vi "Facade.vi"(0 "Data In":T7, 2 "Display State In":T2={"Graph Visible Items"={"Plot Legend"=FALSE, "Scale Legend"=FALSE, "Graph Palette"=FALSE, "Cursor Legend"=FALSE, "X Scrollbar"=FALSE}, "View Table"=FALSE, "Table Visible Items"={"Vertical Scrollbar"=FALSE, "Horizontal Scrollbar"=FALSE, "Row Headers"=FALSE, "Column Headers"=FALSE, "Vertical Lines"=FALSE, "Horizontal Lines"=FALSE}, "Header Font"={"Font Name"="", "Size"=0, "Bold"=FALSE, "Italic"=FALSE, "Underline"=FALSE, "Strikeout"=FALSE, "Color"=0}, "Cell Font"={"Font Name"="", "Size"=0, "Bold"=FALSE, "Italic"=FALSE, "Underline"=FALSE, "Strikeout"=FALSE, "Color"=0}, "Description and Tip..."={"Description"="", "Tip"=""}, "Moveable Splitter Position"=0, "Measurement Cursor Configuration"={"XY"={"enable XY"=FALSE, "Position (X)"=[], "Type"=enum."Absolute", "Y reference"=0.0, "color"=0}, "band"={"enable band"=FALSE, "B1"=0.0, "B2"=0.0, "Fixed bandwidth (B2-B1)"=0.0, "B1 color"=0, "B2 color"=0}, "harmonic"={"enable harmonics"=FALSE, "X reference (1X)"=0.0, "Maximum"=0, "Subset"=enum."All", "1X color"=0, "MX color"=0}, "sideband"={"enable sideband"=FALSE, "X center (C)"=0.0, "Sidebands"=0, "X spacing (s)"=0.0, "Center color"=0, "Sideband color"=0}}, "Cursors"={"List"=[], "Tags"=[]}, "X Increment"=0.0, "X Scale"={"Label Visible"=FALSE, "Label Text"="", "Mapping Mode"=0, "Format String"=""}, "Y Scale"={"Label Visible"=FALSE, "Label Text"="", "Mapping Mode"=0, "Format String"=""}, "Colors"={"background"=16777215, "major grid"=8355711, "minor grid"=12632256, "font"=0}, "desired spectrum view"={"scaling"={"linear/dB"=enum."no change", "dB reference"=0.0, "power/magnitude"=enum."no change", "view"=enum."no change"}, "spectral density"=enum."no change"}, "Plot Color Wheel"=[3381759, 32768, 982784, 4375295, 13827953, 13457919, 16757522, 4343295, 16728758, 12095254], "Plots"=[], "registered user events"=variant, "Lock 1X to Peak"=FALSE, "spectrum component"=32, "phase spectrum view"={"desired units"=0, "desired wrapping"=4}} {"phase spectrum view"."desired wrapping" items=["No change", "Unwrap", "Wrap: -360 to 0", "Wrap: -270 to 90", "Wrap: -180 to 180", "Wrap: -90 to 270", "Wrap: 0 to 360", "Wrap: custom range"]; "phase spectrum view"."desired units" items=["No change", "Radians", "Degrees", "Cycles"]; "spectrum component" items=["Magnitude^2"=37, "Magnitude"=32, "Phase"=33, "Real"=34, "Imaginary"=35, "Coherence"=36, "Unknown"=99]; "Y Scale"."Mapping Mode" items=["Linear", "Logarithmic", "dB"]; "X Scale"."Mapping Mode" items=["Linear", "Logarithmic"]}, 3 "Container State":T6) -> (6 "Data Out":T7, 7 "Display State Out":T2={"Graph Visible Items"={"Plot Legend"=FALSE, "Scale Legend"=FALSE, "Graph Palette"=FALSE, "Cursor Legend"=FALSE, "X Scrollbar"=FALSE}, "View Table"=FALSE, "Table Visible Items"={"Vertical Scrollbar"=FALSE, "Horizontal Scrollbar"=FALSE, "Row Headers"=FALSE, "Column Headers"=FALSE, "Vertical Lines"=FALSE, "Horizontal Lines"=FALSE}, "Header Font"={"Font Name"="", "Size"=0, "Bold"=FALSE, "Italic"=FALSE, "Underline"=FALSE, "Strikeout"=FALSE, "Color"=0}, "Cell Font"={"Font Name"="", "Size"=0, "Bold"=FALSE, "Italic"=FALSE, "Underline"=FALSE, "Strikeout"=FALSE, "Color"=0}, "Description and Tip..."={"Description"="", "Tip"=""}, "Moveable Splitter Position"=0, "Measurement Cursor Configuration"={"XY"={"enable XY"=FALSE, "Position (X)"=[], "Type"=enum."Absolute", "Y reference"=0.0, "color"=0}, "band"={"enable band"=FALSE, "B1"=0.0, "B2"=0.0, "Fixed bandwidth (B2-B1)"=0.0, "B1 color"=0, "B2 color"=0}, "harmonic"={"enable harmonics"=FALSE, "X reference (1X)"=0.0, "Maximum"=0, "Subset"=enum."All", "1X color"=0, "MX color"=0}, "sideband"={"enable sideband"=FALSE, "X center (C)"=0.0, "Sidebands"=0, "X spacing (s)"=0.0, "Center color"=0, "Sideband color"=0}}, "Cursors"={"List"=[], "Tags"=[]}, "X Increment"=0.0, "X Scale"={"Label Visible"=FALSE, "Label Text"="", "Mapping Mode"=0, "Format String"=""}, "Y Scale"={"Label Visible"=FALSE, "Label Text"="", "Mapping Mode"=0, "Format String"=""}, "Colors"={"background"=16777215, "major grid"=8355711, "minor grid"=12632256, "font"=0}, "desired spectrum view"={"scaling"={"linear/dB"=enum."no change", "dB reference"=0.0, "power/magnitude"=enum."no change", "view"=enum."no change"}, "spectral density"=enum."no change"}, "Plot Color Wheel"=[3381759, 32768, 982784, 4375295, 13827953, 13457919, 16757522, 4343295, 16728758, 12095254], "Plots"=[], "registered user events"=variant, "Lock 1X to Peak"=FALSE, "spectrum component"=32, "phase spectrum view"={"desired units"=0, "desired wrapping"=4}} {"phase spectrum view"."desired wrapping" items=["No change", "Unwrap", "Wrap: -360 to 0", "Wrap: -270 to 90", "Wrap: -180 to 180", "Wrap: -90 to 270", "Wrap: 0 to 360", "Wrap: custom range"]; "phase spectrum view"."desired units" items=["No change", "Radians", "Degrees", "Cycles"]; "spectrum component" items=["Magnitude^2"=37, "Magnitude"=32, "Phase"=33, "Real"=34, "Imaginary"=35, "Coherence"=36, "Unknown"=99]; "Y Scale"."Mapping Mode" items=["Linear", "Logarithmic", "dB"]; "X Scale"."Mapping Mode" items=["Linear", "Logarithmic"]}, 8 "Action":T1)   [LabVIEW 2017, in "Spectrum with Cursors.xctl"]
doc: "This is the facade VI for the Spectral Graph with Measurement Cursors XControl.\nThe facade VI is only used within the context of the XControl."
uses:
  <vilib>/addons/_XControls/Spectrum with Cursors/Spectrum with Cursors.xctl
  <vilib>/addons/_XControls/Spectrum with Cursors/Controls/Data.ctl
  <vilib>/addons/_NISVFA/_Shared subVIs/Data Objects/Data/Data.lvclass
  <vilib>/_xctls/Container State.ctl
  <vilib>/addons/_XControls/Spectrum with Cursors/Controls/State.ctl
  <vilib>/Utility/miscctls.llb/LVFontTypeDef.ctl
  <vilib>/addons/_XControls/Spectrum with Cursors/Controls/Measurement Cursor Configuration.ctl
  <vilib>/addons/_NISVFA/_Shared subVIs/Controls/NI Spectrum Component.ctl
  <vilib>/_xctls/Action.ctl
  <vilib>/addons/_NISVFA/_Shared subVIs/Data Objects/Data/Data.lvclass/Data.ctl
  <vilib>/addons/_XControls/Spectrum with Cursors/Controls/Refnums Typedef.ctl
  <vilib>/addons/_NISVFA/_Shared subVIs/Data Objects/Y (DBL)/Y (N Ch).lvclass/Y (N Ch).ctl
  <vilib>/addons/_XControls/Spectrum with Cursors/Controls/Spectrum XControl Events.ctl
  <vilib>/Utility/miscctls.llb/LVForegroundBackgroundColorsTypeDef.ctl
  <vilib>/addons/_NISVFA/_Shared subVIs/Data Objects/Data/Read Channel Count.vi
  <vilib>/addons/_NISVFA/_Shared subVIs/Data Objects/Y (DBL)/SV Convert Spectra to Data Object.vi
  <vilib>/addons/_NISVFA/_Spectrum Processing/SVFA Get Spectrum Subset (1 Ch).vi
  <vilib>/addons/_NISVFA/_Spectrum Processing/SVFA Spectrum Peak Search (1 Ch).vi
  <vilib>/addons/_NISVFA/_Shared subVIs/Data Objects/Data/Read Data Attributes.vi
  <vilib>/addons/_NISVFA/_Shared subVIs/Data Objects/subVIs/Get Channel Count.vi
  <vilib>/addons/_NISVFA/_Shared subVIs/Common/sv_Get NI Property Name String.vi
  <vilib>/addons/_NISVFA/_Shared subVIs/Data Objects/Data/Write Data Attributes.vi
  <vilib>/addons/_NISVFA/_Shared subVIs/Data Objects/subVIs/Set Channel Count.vi
  <vilib>/addons/_NISVFA/_Shared subVIs/Common/svc_Spectrum Units.vi
  <vilib>/addons/_NISVFA/_Spectrum Processing/subVIs/svfa_Spectrum Peak Search.vi
  <vilib>/addons/_NISVFA/_Spectrum Processing/subVIs/svfa_Peak Rough Search Indices.vi
  <vilib>/addons/_NISVFA/_Shared subVIs/Data Objects/Y (DBL)/Y (N Ch).lvclass
  C:/Program Files (x86)/National Instruments/LabVIEW 2017/vi.lib/addons/_NISVFA/_Shared subVIs/Data Objects/Data/Data.lvclass
  <vilib>/addons/_NISVFA/_Spectrum Processing/SVFA Phase Unit Conversion (N Ch).vi
  <vilib>/addons/_NISVFA/_Spectrum Processing/SVFA Wrap or Unwrap Phase (N Ch).vi
  <vilib>/addons/_NISVFA/_Shared subVIs/Common/svc_Caller VI Returned in Error Source.vi
  <vilib>/addons/_NISVFA/_Shared subVIs/Common/svc_Get Weighting Enum and Labels.vi
  <vilib>/addons/_NISVFA/_Shared subVIs/Common/svc_Unit Label Lexical Class.vi
  <vilib>/addons/_NISVFA/_Shared subVIs/Common/svc_Engineering Units to Unit Label.vi
  <vilib>/addons/_NISVFA/_Shared subVIs/Common/svc_Format Value (DBL).vi
  <vilib>/addons/_NISVFA/_Spectrum Processing/subVIs/svfa_Three Finger Peak Search.vi
  <vilib>/addons/_NISVFA/_Shared subVIs/Common/svc_Build Unit Label for Frequency Range.vi
  <vilib>/addons/_NISVFA/_Shared subVIs/Common/svc_Convert Frequency to Frequency String.vi
  <vilib>/addons/_NISVFA/_Shared subVIs/Common/svc_Check Frequency Range in Spectrum.vi
  <vilib>/addons/_NISVFA/_Spectrum Processing/SVFA Unit Conversion (N Ch).vi
  <vilib>/addons/_NISVFA/_Shared subVIs/Spectrum Info/sv_Convert Spectrum Info to Variant Attributes.vi
  <vilib>/addons/_NISVFA/_Shared subVIs/Data Objects/Y (DBL)/Write Channels Array.vi
  <vilib>/_xctls/XControlSupport.lvlib
panel:
  out "plot names":string[](array[string])
  in  "Focus Boolean":bool
  out "Spectra Graph":cluster{"x0":dbl, "dx":dbl, "magnitude":dbl[]}[](graph)
  in  "View Table":bool=TRUE
  in  "Cursor Table":string[][](table)
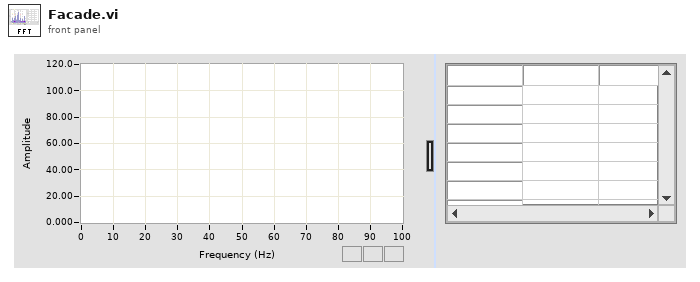
[diagram p1: front panel]
types:
  T1 = typedef "XControlSupport.lvlib/Action.ctl" = cluster{"Data Changed?":bool, "State Changed?":bool, "Action Name":string}
  T2 = typedef "Spectrum with Cursors.xctl/State.ctl" = cluster{"Graph Visible Items":cluster{"Plot Legend":bool, "Scale Legend":bool, "Graph Palette":bool, "Cursor Legend":bool, "X Scrollbar":bool}, "View Table":bool, "Table Visible Items":cluster{"Vertical Scrollbar":bool, "Horizontal Scrollbar":bool, "Row Headers":bool, "Column Headers":bool, "Vertical Lines":bool, "Horizontal Lines":bool}, "Header Font":T3, "Cell Font":T3, "Description and Tip...":cluster{"Description":string, "Tip":string}, "Moveable Splitter Position":i32, "Measurement Cursor Configuration":T4, "Cursors":cluster{"List":cluster{"Name":string, "Color":u32, "Style":i32, "Point Style":u8, "Name Visible":bool, "Allow Drag":bool, "Cursor Mode":u32, "Plot":i32, "Index":i32, "Position":cluster{"X":dbl, "Y":dbl}, "X Scale":u32, "Y Scale":u32, "Watch Plots":i32[], "Watch All Plots":bool, "Plot Area":i32, "Label Offset":cluster{"X":dbl, "Y":dbl}}[], "Tags":variant[]}, "X Increment":dbl, "X Scale":cluster{"Label Visible":bool, "Label Text":string, "Mapping Mode":u8, "Format String":string}, "Y Scale":cluster{"Label Visible":bool, "Label Text":string, "Mapping Mode":u8, "Format String":string}, "Colors":cluster{"background":u32, "major grid":u32, "minor grid":u32, "font":u32}, "desired spectrum view":cluster{"scaling":cluster{"linear/dB":enum16{"no change", "linear", "dB"}, "dB reference":dbl, "power/magnitude":enum16{"no change", "power", "magnitude"}, "view":enum16{"no change", "rms", "peak", "peak-peak"}}, "spectral density":enum16{"no change", "spectrum", "spectral density"}}, "Plot Color Wheel":u32[], "Plots":cluster{"Name":string, "Line Color":u32, "Line Style":u8, "Line Width":u8, "Fill/Point Color":u32, "Point Style":u8, "Fill To":i16, "Interpolation":u8, "Anti-aliased":bool}[], "registered user events":variant, "Lock 1X to Peak":bool, "spectrum component":T5, "phase spectrum view":cluster{"desired units":u16, "desired wrapping":u16}}
  T3 = typedef "LVFontTypeDef.ctl" = cluster{"Font Name":string, "Size":u16, "Bold":bool, "Italic":bool, "Underline":bool, "Strikeout":bool, "Color":u32}
  T4 = typedef "Spectrum with Cursors.xctl/Measurement Cursor Configuration.ctl" = cluster{"XY":cluster{"enable XY":bool, "Position (X)":dbl[], "Type":enum16{"Absolute", "Relative"}, "Y reference":dbl, "color":u32}, "band":cluster{"enable band":bool, "B1":dbl, "B2":dbl, "Fixed bandwidth (B2-B1)":dbl, "B1 color":u32, "B2 color":u32}, "harmonic":cluster{"enable harmonics":bool, "X reference (1X)":dbl, "Maximum":i32, "Subset":enum16{"All", "Even", "Odd"}, "1X color":u32, "MX color":u32}, "sideband":cluster{"enable sideband":bool, "X center (C)":dbl, "Sidebands":i32, "X spacing (s)":dbl, "Center color":u32, "Sideband color":u32}}
  T5 = typedef "NI Spectrum Component.ctl" = u16
  T6 = typedef "XControlSupport.lvlib/Container State.ctl" = cluster{"Indicator?":bool, "Run Mode?":bool, " Refnum":refnum<vi>}
  T7 = typedef "Spectrum with Cursors.xctl/Data.ctl" = refnum<class "Data.lvclass">
  T8 = typedef "Spectrum with Cursors.xctl/Refnums Typedef.ctl" = cluster{"Facade Panel Refnum":refnum<vi>, "Splitters":cluster{"Moveable":refnum<vi>, "Locked":refnum<vi>}, "Panes":cluster{"Container":refnum<vi>, "Graph":refnum<vi>, "Table":refnum<vi>, "Fixed-Width":refnum<vi>}, "Controls":cluster{"Graph":refnum<vi>, "Table":refnum<vi>, "View Table":refnum<vi>, "Focus Boolean":refnum<vi>, "Plot Names":refnum<vi>}}
  T9 = enum16{"no change", "spectrum", "spectral density"}
  T10 = cluster{"single/multiple":enum16{"Multiple Peaks", "Single Max Peak"}, "threshold":dbl}
  T11 = enum16{"No change", "Unwrap", "Wrap: -360 to 0", "Wrap: -270 to 90", "Wrap: -180 to 180", "Wrap: -90 to 270", "Wrap: 0 to 360", "Wrap: custom range"}
  T12 = enum16{"No change", "Radians", "Degrees", "Cycles"}
  T13 = typedef "Spectrum with Cursors.xctl/Spectrum XControl Events.ctl" = string
  T14 = typedef "LVForegroundBackgroundColorsTypeDef.ctl" = cluster{"Foreground Color":u32, "Background Color":u32}
  T15 = typedef "svc_Spectrum Info.ctl" = cluster{"channel name":string, "description":string, "x-axis units":T16, "spectral info":cluster{"spectrum type":T17, "linear/dB":enum16{"linear", "dB"}, "window":u16, "window size":i32, "FFT size":i32}, "engineering units":T18, "custom label":string, "dB reference [EU]":dbl, "peak units":enum16{"rms", "peak", "peak-peak"}, "weighting filter":T19, "spectral density?":bool, "unit label":string, "spectrum skewed?":bool, "complimentary spectrum units":T20}
  T16 = typedef "svc_X-Axis Units.ctl" = u16
  T17 = typedef "svc_Spectrum Type.ctl" = enum16{"FFT Spectrum [complex]", "Amplitude [Magnitude]", "Power [Magnitude^2]", "Cross Spectrum [complex]", "Frequency Response [Complex]"}
  T18 = typedef "svc_Engineering Units Text Ring.ctl" = u16
  T19 = typedef "svc_Weighting Filter Text Ring.ctl" = u16
  T20 = typedef "svc_Complimentary Spectrum Units.ctl" = enum16{"none", "radians", "degrees", "cycles", "imaginary"}
  T21 = typedef "eventvkey.ctl" = enum16{"ASCII", "Enter", "Return", "Shift", "Ctrl", "Alt", "Cmd", "Opt", "Caps", "NumLock", "Clear", "Break", "Up", "Down", "Left", "Right", "Insert", "Delete", "Home", "End", "PageUp", "PageDown", "Escape", "Help", "Pause", "ScrollLock", "F1", "F2", "F3", "F4", "F5", "F6", "F7", "F8", "F9", "F10", "F11", "F12", "F13", "F14", "F15", "F16", "F17", "F18", "F19", "F20", "F21", "F22", "F23", "F24", "Play", "VolumeUp", "VolumeDown", "Mute", "Two Byte Char"}
  T22 = cluster{"Shift":bool, "Ctrl":bool, "Alt":bool, "Cmd":bool, "Opt":bool}
  T23 = cluster{"linear/dB":enum16{"no change", "linear", "dB"}, "dB reference":dbl, "power/magnitude":enum16{"no change", "power", "magnitude"}, "view":enum16{"no change", "rms", "peak", "peak-peak"}}
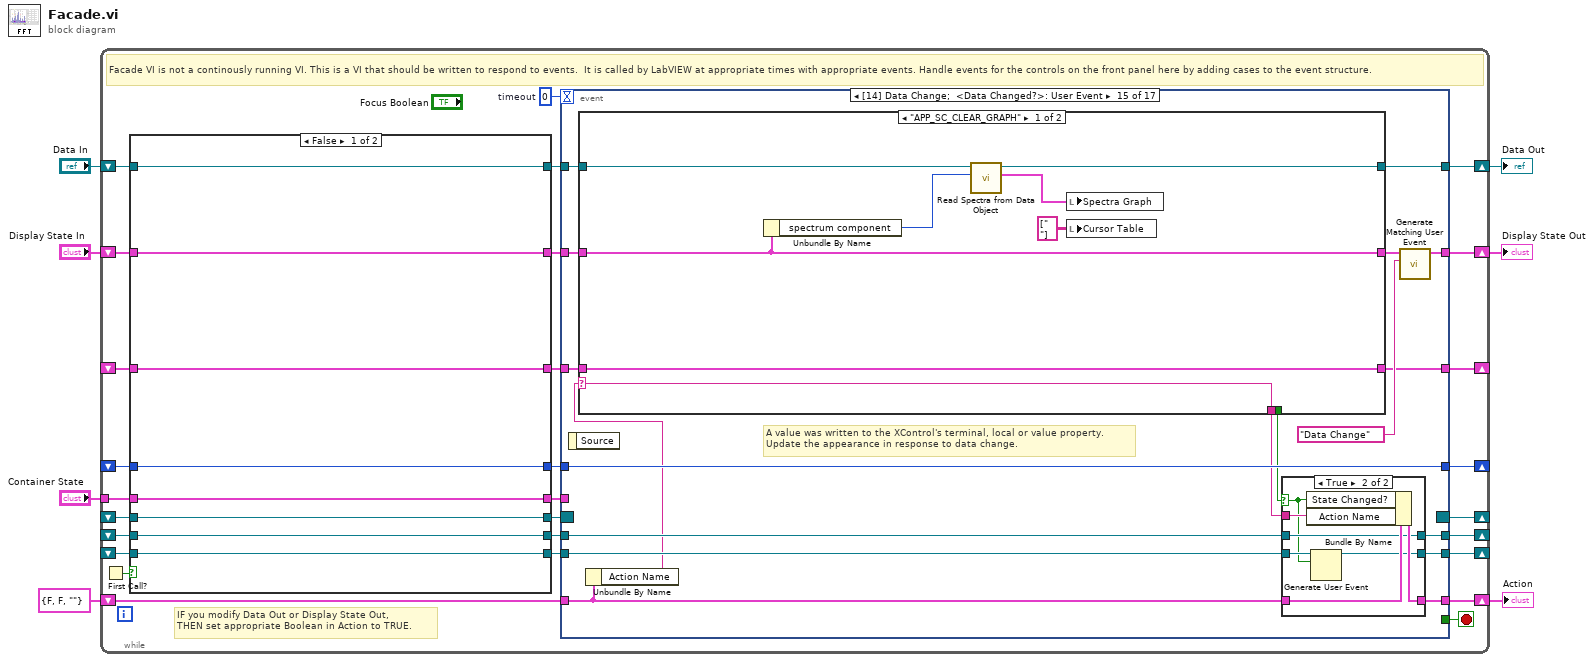
[diagram p0: block diagram]
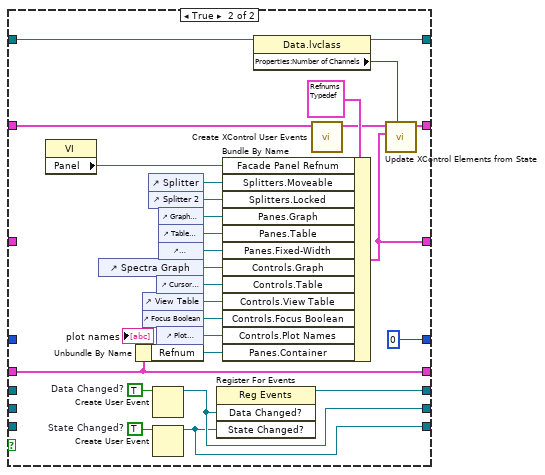
[diagram p2: hidden frame]
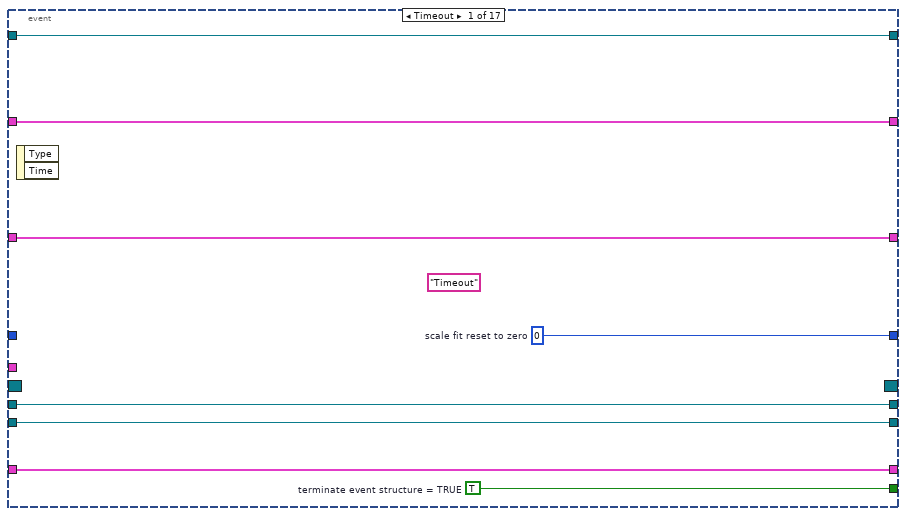
[diagram p3: hidden frame]
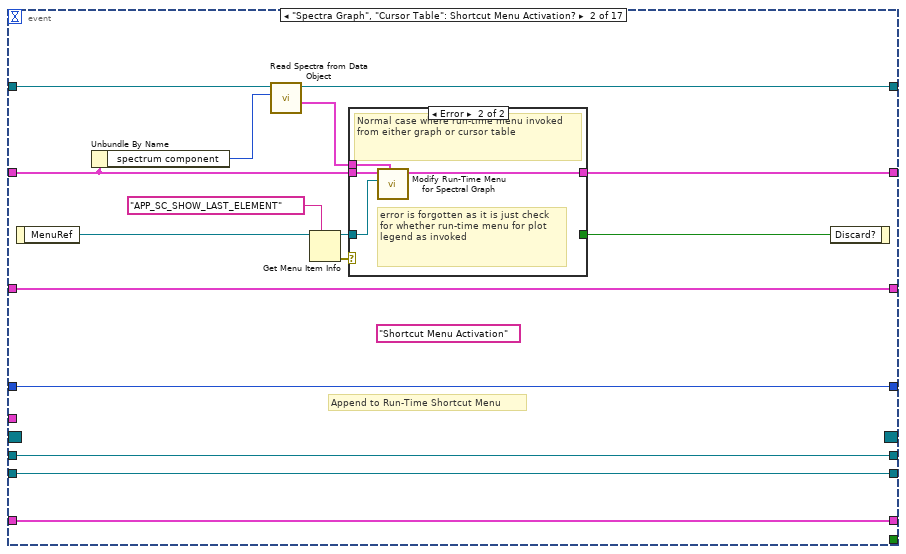
[diagram p4: hidden frame]
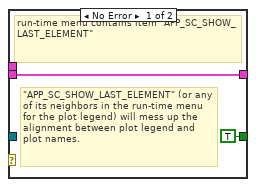
[diagram p5: hidden frame]
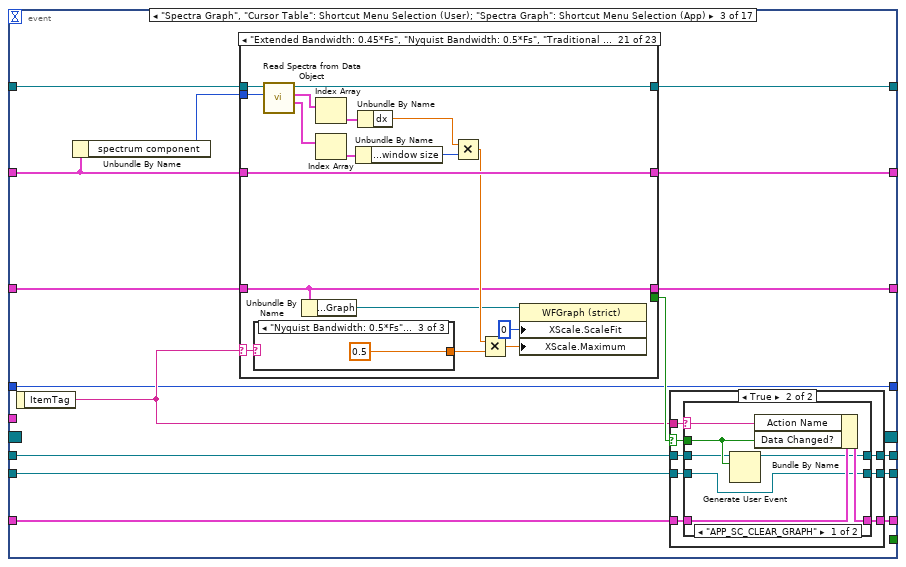
[diagram p6: hidden frame]
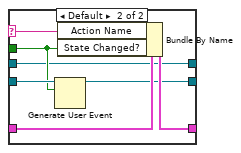
[diagram p8: hidden frame]
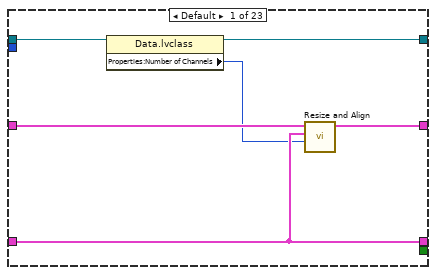
[diagram p9: hidden frame]
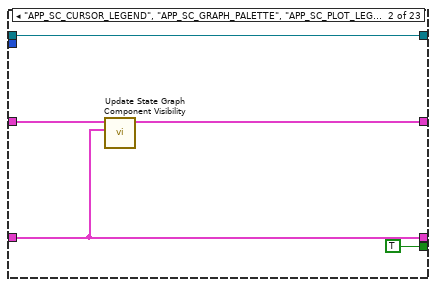
[diagram p10: hidden frame]
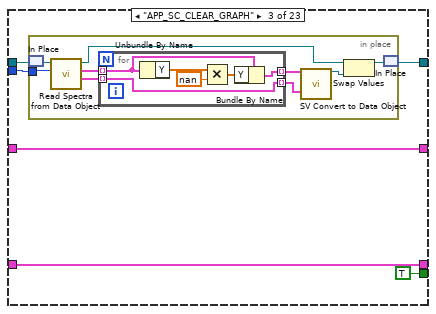
[diagram p11: hidden frame]
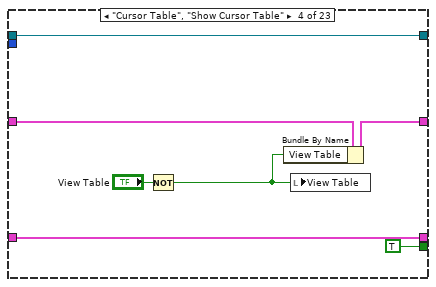
[diagram p12: hidden frame]
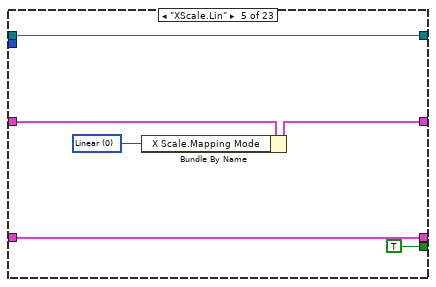
[diagram p13: hidden frame]
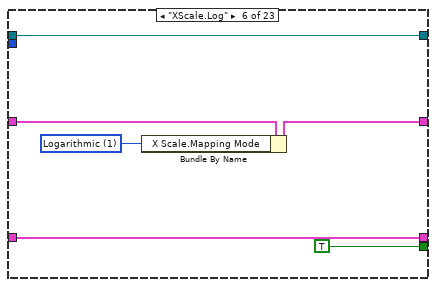
[diagram p14: hidden frame]
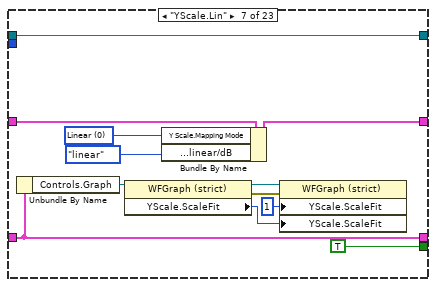
[diagram p15: hidden frame]
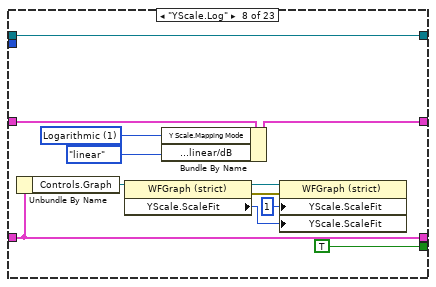
[diagram p16: hidden frame]
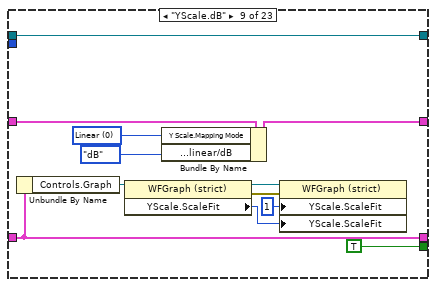
[diagram p17: hidden frame]
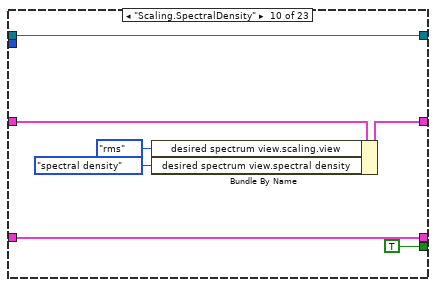
[diagram p18: hidden frame]
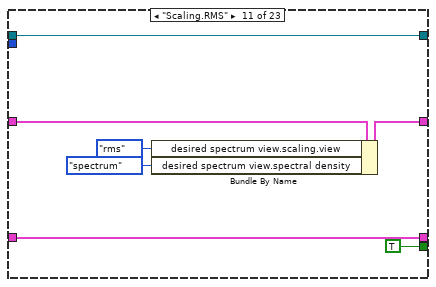
[diagram p19: hidden frame]
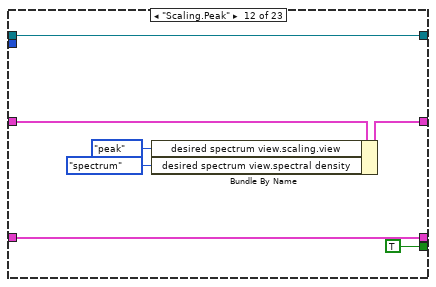
[diagram p20: hidden frame]
diagram:
  n1 = while {
    shift-right: [w30] -> w5
    shift-left: "Display State In" -> [w14]
    tunnel: "Container State" -> [w20]
    shift-right: [w33] -> w7
    shift-left: "Data In" -> [w9]
    shift-right: [w31] -> w2
    shift-left: T1 {"Data Changed?"=FALSE, "State Changed?"=FALSE, "Action Name"=""} ("Action") -> [w32]
    shift-right: [w27] -> _
    shift-left: _ -> [w25]
    shift-right: [w22] -> _
    shift-left: _ -> [w21]
    shift-right: [w26] -> _
    shift-left: _ -> [w23]
    shift-right: [w15] -> _
    shift-left: _ -> [w17]
    shift-right: [w12] -> _
    shift-left: _ -> [w11]
    stop <- w35 stop-if-true
    w34 = 0  # timeout
    # "IF you modify Data Out or Display State Out, \nTHEN set appropriate Boolean in Action to TRUE."
    # "Facade VI is not a continously running VI. This is a VI that should be written to respond to events.  It is called by LabVIEW at appropriate times with appropriate events. Handle events for the controls on the front panel here by adding cases to the event structure."
    n2 = First Call?() -> (First Call?: T/F=w24:bool)
    n3 = case shown="False" w24 {
      tunnel: [w43 w57] -> w16
      tunnel: [w42 w58] -> w29
      tunnel: [w41 w59] -> w28
      tunnel: w25 -> [w43 _]
      tunnel: w23 -> [w42 _]
      tunnel: w21 -> [w41 _]
      tunnel: w20 -> [w39 w53]
      tunnel: [w39 w53] -> w19
      tunnel: [w40 w49] -> w18
      tunnel: w17 -> [w40 _]
      tunnel: w14 -> [w37 w52]
      tunnel: [w37 w50] -> w13
      tunnel: [w38 u8 0 ("Scale Fit")] -> w10
      tunnel: w11 -> [w38 _]
      tunnel: w9 -> [w36 w46]
      tunnel: [w36 w45] -> w8
      frame False {
      }
      frame True {
        w70 = TRUE  # State Changed?
        w69 = TRUE  # Data Changed?
        n4 = property class="VI"() -> ("Panel"=w48:refnum<vi>)  [unwired: 2 in, 2 out]
        n5 = control-ref of="Spectra Graph"() -> (w65:refnum<vi>)
        n6 = Unbundle By Name(w53) -> ("Refnum"=w55:refnum<vi>)
        n7 = control-ref of="View Table"() -> (w63:refnum<vi>)
        n8 = control-ref of="Focus Boolean"() -> (w56:refnum<vi>)
        n9 = control-ref of="Splitter"() -> (w62:refnum<vi>)
        n10 = control-ref of="Splitter 2"() -> (w61:refnum<vi>)
        n11 = Create User Event(user event datatype=w69) -> (user event=w59:refnum<user-event>)  [unwired: 1 in, 1 out]
        n12 = Create User Event(user event datatype=w70) -> (user event=w58:refnum<user-event>)  [unwired: 1 in, 1 out]
        n13 = control-ref of="Cursor Table"() -> (w64:refnum<vi>)
        n14 = control-ref of="Plot Names"() -> (w54:refnum<vi>)
        n15 = control-ref of="Graph Pane"() -> (w60:refnum<vi>)
        n16 = control-ref of="Table Pane"() -> (w67:refnum<vi>)
        n17 = control-ref of="Fixed-Width Pane"() -> (w66:refnum<vi>)
        n18 = register-events(w59, w58) -> (reference out=w57:refnum<event-registration>)  [unwired: 2 in, 1 out]
        n19 = Bundle By Name(cluster=T8 {"Facade Panel Refnum"=refnum, "Splitters"={"Moveable"=refnum, "Locked"=refnum}, "Panes"={"Container"=refnum, "Graph"=refnum, "Table"=refnum, "Fixed-Width"=refnum}, "Controls"={"Graph"=refnum, "Table"=refnum, "View Table"=refnum, "Focus Boolean"=refnum, "Plot Names"=refnum}} ("Refnums for Resizing and Alignment"), "Facade Panel Refnum"=w48, "Splitters.Moveable"=w62, "Splitters.Locked"=w61, "Panes.Graph"=w60, "Panes.Table"=w67, "Panes.Fixed-Width"=w66, "Controls.Graph"=w65, "Controls.Table"=w64, "Controls.View Table"=w63, "Controls.Focus Boolean"=w56, "Controls.Plot Names"=w54, "Panes.Container"=w55) -> (w49:T8)
        n20 = property class="Data.lvclass"(reference=w46) -> (reference out=w45:T7, "Properties:Number of Channels"=w44:i32)  [unwired: 1 in, 1 out]
        n21 = call <vilib>:"Create XControl User Events.vi"("Display State In in"=w52) -> ("Display State In out"=w47:T2)  [unwired: 9 in, 1 out]
        n22 = call <vilib>:"Update XControl Elements from State.vi"("number of channels"=w44, "Refnums for FP Objects"=w49, "State in"=w47) -> ("State out"=w50:T2)  [unwired: 8 in]
      }
    }
    n23 = event shown="[14] Data Change;  <Data Changed?>: User Event" {
      selector: w16 -> [_ _ _ _ _ _ _ _ _ _ _ _ _ _ _ _ _]
      dyn-events: [_ _ _ _ _ _ _ _ _ _ _ _ _ _ _ _ _] -> w27
      timeout: w34 -> [_ _ _ _ _ _ _ _ _ _ _ _ _ _ _ _ _]
      tunnel: w13 -> [w76 w80 w102 w411 w437 w448 w479 w514 w529 w542 w587 w628 w666 w685 w721 w893 w901]
      tunnel: [w76 w90 w116 w408 w436 w447 w478 w497 w528 w545 w589 w630 w665 w686 w729 w893 w901] -> w30
      tunnel: [w78 _ _ _ _ _ _ _ _ _ _ _ _ _ _ _ _] -> w35
      tunnel: w19 -> [_ _ _ _ _ _ _ _ _ _ _ _ _ _ _ w894 w902]
      tunnel: w8 -> [w75 w83 w103 w429 w446 w457 w483 w515 w533 w554 w597 w638 w671 w674 w735 w892 w900]
      tunnel: [w75 w82 w104 w429 w446 w457 w483 w515 w533 w554 w597 w638 w671 w673 w734 w892 w900] -> w33
      tunnel: [w77 w94 w114 w425 w441 w456 w482 w512 w532 w552 w595 w636 w670 w679 w724 w891 w899] -> w31
      tunnel: w32 -> [w77 w94 w115 w426 w442 w456 w482 w513 w532 w553 w596 w637 w670 w680 w719 w891 w899]
      tunnel: w18 -> [w72 w91 w109 w412 w445 w450 w480 w502 w527 w540 w585 w627 w667 w684 w728 w884 w896]
      tunnel: w28 -> [w74 w93 w110 w424 w440 w454 w475 w507 w530 w548 w591 w632 w668 w689 w726 w888 w898]
      tunnel: w29 -> [w73 w92 w113 w423 w439 w455 w474 w510 w531 w551 w594 w635 w669 w677 w725 w887 w897]
      tunnel: [w73 w92 w112 w422 w438 w455 w474 w509 w531 w550 w593 w634 w669 w676 w723 w887 w897] -> w26
      tunnel: [w74 w93 w111 w424 w440 w454 w475 w508 w530 w549 w592 w633 w668 w688 w722 w888 w898] -> w22
      tunnel: [w72 w91 w108 w412 w445 w449 w480 w502 w527 w540 w585 w627 w667 w682 w731 w884 w896] -> w15
      tunnel: [w71 w89 w105 w409 w434 w451 w472 w499 w526 w534 w578 w619 w660 w681 w733 w883 w895] -> w12
      tunnel: w10 -> [_ w89 w105 w409 w434 _ w473 w499 w526 w534 w578 w619 w660 w681 w733 w883 w895]
      event Timeout {
        w71 = u8 0  # scale fit reset to zero
        (unwired) "Timeout"
        w78 = TRUE  # terminate event structure = TRUE
        n24 = event-data() -> ()  [unwired: 1 in, 2 out]
      }
      event "Spectra Graph", "Cursor Table": Shortcut Menu Activation? {
        (unwired) "Shortcut Menu Activation"
        # "Append to Run-Time Shortcut Menu"
        n25 = event-data() -> ("MenuRef"=w88:refnum<k9>)  [unwired: 1 in]
        n26 = Unbundle By Name(w80) -> ("spectrum component"=w79:T5)
        n27 = call-dynamic "Read Spectra from Data Object.vi"("component"=w79, "Data in"=w83) -> ("spectra info"=w81:T15[], "Data out"=w82:T7)  [unwired: 5 in, 3 out]
        n28 = Get Menu Item Info(7:"APP_SC_SHOW_LAST_ELEMENT", 11:w88) -> (0:w85:errorcluster, 3:w87:refnum<k9>)  [unwired: 1 in, 5 out]
        n29 = case shown="Error" w85 {
          tunnel: w80 -> [w96 w100]
          tunnel: [w96 w99] -> w90
          tunnel: w87 -> [_ w98]
          tunnel: [TRUE _] -> w84
          tunnel: w81 -> [_ w97]
          frame No Error {
            # "\"APP_SC_SHOW_LAST_ELEMENT\" (or any of its neighbors in the run-time menu for the plot legend) will mess up the alignment between plot legend and plot names."
            # "run-time menu contains item \"APP_SC_SHOW_LAST_ELEMENT\""
          }
          frame Error {
            # "error is forgotten as it is just check for whether run-time menu for plot legend as invoked"
            # "Normal case where run-time menu invoked from either graph or cursor table"
            n30 = call <vilib>:"Modify Run-Time Menu for Spectral Graph.vi"("spectra info"=w97, "Menu in"=w98, "Display State In"=w100) -> ("Display State out"=w99:T2)  [unwired: 8 in]
          }
        }
        n31 = event-data("Discard?"=w84) -> ()  [unwired: 1 in, 1 out]
      }
      event "Spectra Graph", "Cursor Table": Shortcut Menu Selection (User); "Spectra Graph": Shortcut Menu Selection (App) {
        n32 = event-data() -> ("ItemTag"=w106:string)  [unwired: 1 in]
        n33 = Unbundle By Name(w102) -> ("spectrum component"=w101:T5)
        n34 = case shown="\"Extended Bandwidth: 0.45*Fs\", \"Nyquist Bandwidth: 0.5*Fs\", \"Traditional Bandwidth: 0.39*Fs\"" w106 {
          selector: w106 -> [_ _ _ _ _ _ _ _ _ _ _ _ _ _ _ _ _ _ _ _ w380 w386 w401]
          tunnel: w102 -> [w147 w152 w158 w178 w185 w192 w204 w216 w228 w234 w241 w248 w255 w261 w267 w274 w284 w305 w338 w356 w381 w388 w400]
          tunnel: [w146 w151 w158 w177 w184 w191 w203 w215 w227 w233 w240 w247 w254 w260 w266 w272 w285 w306 w339 w355 w381 w387 w399] -> w116
          tunnel: [_ TRUE ("state changed") TRUE ("state changed") TRUE ("state changed") TRUE ("state changed") TRUE ("state changed") TRUE ("state changed") TRUE ("state changed") TRUE ("state changed") TRUE ("state changed") TRUE ("state changed") TRUE ("state changed") TRUE ("state changed") TRUE ("state changed") TRUE ("state changed") w271 TRUE ("state changed") w294 w331 TRUE ("state changed") _ TRUE ("state changed") TRUE ("state changed")] -> w107
          tunnel: w109 -> [w145 w150 w157 w180 w186 w188 w194 w206 w218 w235 w242 w249 w256 w262 w268 w270 w286 w299 w336 w364 w375 w391 w403]
          tunnel: [w145 w150 w157 w180 w186 w188 w194 w206 w218 w235 w242 w249 w256 w262 w268 w270 w286 w299 w336 w364 w375 w391 w403] -> w108
          tunnel: [w143 w148 w153 w174 w181 w187 w193 w205 w217 w229 w236 w243 w250 w257 w263 w269 w280 w290 w327 w353 w368 w390 w402] -> w104
          tunnel: w103 -> [w144 w148 w154 w174 w181 w187 w193 w205 w217 w229 w236 w243 w250 w257 w263 w269 w280 w291 w328 w353 w369 w390 w402]
          tunnel: w101 -> [_ _ w155 _ _ _ _ _ _ _ _ _ _ _ _ _ _ w287 w324 _ w365 _ _]
          frame Default {
            n35 = property class="Data.lvclass"(reference=w144) -> (reference out=w143:T7, "Properties:Number of Channels"=w142:i32)  [unwired: 1 in, 1 out]
            n36 = call <vilib>:"Resize and Align.vi"("number of channels"=w142, "Refnums for Resizing and Alignment"=w145, "State in"=w147) -> ("State out"=w146:T2)  [unwired: 7 in, 1 out]
          }
          frame "APP_SC_CURSOR_LEGEND", "APP_SC_GRAPH_PALETTE", "APP_SC_PLOT_LEGEND", "APP_SC_SCALE_LEGEND", "APP_SC_X_SCALE", "APP_SC_X_SCROLLBAR", "APP_SC_Y_SCALE" {
            n37 = call <vilib>:"Update State Graph Component Visibility.vi"("Refnums for FP Objects"=w150, "State in"=w152) -> ("State out"=w151:T2)  [unwired: 9 in]
          }
          frame "APP_SC_CLEAR_GRAPH" {
            n38 = in-place {
              in-place-border: w155 -> [w163]
              n39 = in-place-match #1(w154) -> (w162:T7)
              n40 = call-dynamic "Read Spectra from Data Object.vi"("component"=w163, "Data in"=w162) -> ("spectra info"=w166:T15[], "spectra"=w167:cluster{"x0":dbl, "dx":dbl, "Y":dbl[]}[], "Data out"=w159:T7)  [unwired: 5 in, 2 out]
              n41 = for {
                tunnel: w167 -> [w171] mode=indexing
                tunnel: w166 -> [w169] mode=indexing
                tunnel: [w168] -> w165 mode=indexing
                tunnel: [w169] -> w164 mode=indexing
                n42 = Unbundle By Name(w171) -> ("Y"=w173:dbl[])
                n43 = Multiply(x=w173, y=nan) -> (x*y=w170:dbl[])
                n44 = Bundle By Name(cluster=w171, "Y"=w170) -> (w168:cluster{"x0":dbl, "dx":dbl, "Y":dbl[]})
              }
              n45 = call-poly <vilib>:"SV Convert to Data Object.vi"("spectra"=w165, "spectra info"=w164) -> ("Spectrum Data"=w161:refnum<class "Data.lvclass">)  [unwired: 16 in, 1 out]
              n46 = Swap Values(12:w159, 14:w161) -> (1:w160:T7)  [unwired: 1 in, 1 out]
              n47 = in-place-match #1(w160) -> (w153:T7)
            }
          }
          frame "Cursor Table", "Show Cursor Table" {
            n48 = Not(x="View Table") -> (.not. x?=w176:bool)
            n49 = Bundle By Name(cluster=w178, "View Table"=w176) -> (w177:T2)
            n50 = local write "View Table"(w176) -> ()
          }
          frame "XScale.Lin" {
            w182 = u8 0 items=["Linear", "Logarithmic"] ("Mapping Mode")
            n51 = Bundle By Name(cluster=w185, "X Scale.Mapping Mode"=w182) -> (w184:T2)
          }
          frame "XScale.Log" {
            w190 = u8 1 items=["Linear", "Logarithmic"] ("Mapping Mode")
            n52 = Bundle By Name(cluster=w192, "X Scale.Mapping Mode"=w190) -> (w191:T2)
          }
          frame "YScale.Lin" {
            w202 = u8 0 items=["Linear", "Logarithmic"] ("Mapping Mode")
            n53 = Unbundle By Name(w194) -> ("Controls.Graph"=w195:refnum<vi>)
            n54 = property class="WFGraph (strict)"(reference=w195) -> (reference out=w196:refnum<vi>, error out=w197:errorcluster, "YScale.ScaleFit"=w198:u8)  [unwired: 1 in]
            n55 = Bundle By Name(cluster=w204, "Y Scale.Mapping Mode"=w202, "desired spectrum view.scaling.linear/dB"=enum16{"no change", "linear", "dB"}."linear" ("spectrum view.desired scaling.linear/dB")) -> (w203:T2)
            n56 = property class="WFGraph (strict)"(reference=w196, error in=w197, "YScale.ScaleFit"=u8 1 ("Y Scale.Scale Fit"), "YScale.ScaleFit"=w198) -> ()  [unwired: 2 out]
          }
          frame "YScale.Log" {
            w213 = u8 1 items=["Linear", "Logarithmic"] ("Mapping Mode")
            n57 = Unbundle By Name(w206) -> ("Controls.Graph"=w207:refnum<vi>)
            n58 = property class="WFGraph (strict)"(reference=w207) -> (reference out=w208:refnum<vi>, error out=w209:errorcluster, "YScale.ScaleFit"=w210:u8)  [unwired: 1 in]
            n59 = Bundle By Name(cluster=w216, "Y Scale.Mapping Mode"=w213, "desired spectrum view.scaling.linear/dB"=enum16{"no change", "linear", "dB"}."linear" ("spectrum view.desired scaling.linear/dB")) -> (w215:T2)
            n60 = property class="WFGraph (strict)"(reference=w208, error in=w209, "YScale.ScaleFit"=u8 1 ("Y Scale.Scale Fit"), "YScale.ScaleFit"=w210) -> ()  [unwired: 2 out]
          }
          frame "YScale.dB" {
            w225 = u8 0 items=["Linear", "Logarithmic"] ("Mapping Mode")
            n61 = Unbundle By Name(w218) -> ("Controls.Graph"=w219:refnum<vi>)
            n62 = property class="WFGraph (strict)"(reference=w219) -> (reference out=w220:refnum<vi>, error out=w221:errorcluster, "YScale.ScaleFit"=w222:u8)  [unwired: 1 in]
            n63 = Bundle By Name(cluster=w228, "Y Scale.Mapping Mode"=w225, "desired spectrum view.scaling.linear/dB"=enum16{"no change", "linear", "dB"}."dB" ("spectrum view.desired scaling.linear/dB")) -> (w227:T2)
            n64 = property class="WFGraph (strict)"(reference=w220, error in=w221, "YScale.ScaleFit"=u8 1 ("Y Scale.Scale Fit"), "YScale.ScaleFit"=w222) -> ()  [unwired: 2 out]
          }
          frame "Scaling.SpectralDensity" {
            n65 = Bundle By Name(cluster=w234, "desired spectrum view.scaling.view"=enum16{"no change", "rms", "peak", "peak-peak"}."rms", "desired spectrum view.spectral density"=T9."spectral density") -> (w233:T2)
          }
          frame "Scaling.RMS" {
            n66 = Bundle By Name(cluster=w241, "desired spectrum view.scaling.view"=enum16{"no change", "rms", "peak", "peak-peak"}."rms", "desired spectrum view.spectral density"=T9."spectrum") -> (w240:T2)
          }
          frame "Scaling.Peak" {
            n67 = Bundle By Name(cluster=w248, "desired spectrum view.scaling.view"=enum16{"no change", "rms", "peak", "peak-peak"}."peak", "desired spectrum view.spectral density"=T9."spectrum") -> (w247:T2)
          }
          frame "Scaling.Peak-Peak" {
            n68 = Bundle By Name(cluster=w255, "desired spectrum view.scaling.view"=enum16{"no change", "rms", "peak", "peak-peak"}."peak-peak", "desired spectrum view.spectral density"=T9."spectrum") -> (w254:T2)
          }
          frame "Scaling.Magnitude" {
            n69 = Bundle By Name(cluster=w261, "desired spectrum view.scaling.power/magnitude"=enum16{"no change", "power", "magnitude"}."magnitude") -> (w260:T2)
          }
          frame "Scaling.Power" {
            n70 = Bundle By Name(cluster=w267, "desired spectrum view.scaling.power/magnitude"=enum16{"no change", "power", "magnitude"}."power") -> (w266:T2)
          }
          frame "Configure Cursors..." {
            n71 = call <vilib>:"Configure Measurement Cursors.vi"("State in"=w274) -> ("OK"=w271:bool, "State out"=w273:T2)  [unwired: 9 in]
            n72 = case shown="True" w271 {
              tunnel: w273 -> [w275 w279]
              tunnel: [w275 w277] -> w272
              tunnel: w270 -> [_ w276]
              frame False {
              }
              frame True {
                n73 = call <vilib>:"Update Cursors from Measurement Cursor Configuration.vi"("State in"=w279) -> ("State out"=w278:T2)  [unwired: 10 in]
                n74 = call <vilib>:"Update Graph Cursors from State.vi"("Refnums for FP Objects"=w276, "State in"=w278) -> ("State out"=w277:T2)  [unwired: 9 in]
              }
            }
          }
          frame "Lock 1X to Peak" {
            n75 = Unbundle By Name(w284) -> ("Lock 1X to Peak"=w283:bool)
            n76 = Not(x=w283) -> (.not. x?=w282:bool)
            n77 = Bundle By Name(cluster=w284, "Lock 1X to Peak"=w282) -> (w285:T2)
          }
          frame "Snap 1X to Peak" {
            n78 = Unbundle By Name(w305) -> ("Measurement Cursor Configuration.harmonic.X reference (1X)"=w303:dbl)
            n79 = Unbundle By Name(w299) -> ("Controls.Table"=w298:refnum<vi>)
            n80 = call-dynamic "Read Spectra from Data Object.vi"("component"=w287, "Data in"=w291) -> ("spectra info"=w292:T15[], "spectra"=w293:cluster{"x0":dbl, "dx":dbl, "Y":dbl[]}[], "Data out"=w290:T7)  [unwired: 5 in, 2 out]
            n81 = Index Array(array=w293) -> (element=w289:cluster{"x0":dbl, "dx":dbl, "Y":dbl[]})  [unwired: 1 in]
            n82 = Index Array(array=w292) -> (element=w288:T15)  [unwired: 1 in]
            n83 = property class="Tbl"(reference=w298) -> (reference out=w297:refnum<vi>, "Key Focus"=w296:bool)  [unwired: 1 in, 1 out]
            n84 = Multiply(x=cluster{"start":dbl, "stop":dbl} {"start"=0.5, "stop"=1.5} ("range"), y=w303) -> (x*y=w301:cluster{"start":dbl, "stop":dbl})
            n85 = call-poly <vilib>:"SVFA Get Spectrum Subset.vi"("spectrum"=w289, "range"=w301, "spectrum info"=w288) -> ("spectrum subset"=w310:cluster{"x0":dbl, "dx":dbl, "magnitude":dbl[]}, "dup spectrum info"=w308:T15, "error out"=w307:errorcluster)  [unwired: 11 in, 3 out]
            n86 = call-poly <vilib>:"SVFA Spectrum Peak Search.vi"("spectrum"=w310, "peak search settings"=T10 {"single/multiple"=enum."Single Max Peak", "threshold"=inf}, "spectrum info in"=w308, "error in (no error)"=w307) -> ("peaks"=w304:cluster{"freq. or order":dbl, "value":dbl}[], "number of peaks"=w300:i32)  [unwired: 11 in, 3 out]
            n87 = case shown="1" w300 {
              tunnel: [w315 w323] -> w306
              tunnel: w305 -> [w315 w322]
              tunnel: w304 -> [_ w321]
              tunnel: w299 -> [_ w318]
              tunnel: [_ w316] -> w294
              frame 0, Default {
              }
              frame 1 {
                n88 = Index Array(array=w321) -> (element=w320:cluster{"freq. or order":dbl, "value":dbl})  [unwired: 1 in]
                n89 = Unbundle By Name(w320) -> ("freq. or order"=w319:dbl)
                n90 = call <vilib>:"Move Set on Cursor Move.vi"("Cursor.Position.X"=w319, "Cursor Name"="1X", "Refnums for Resizing and Alignment"=w318, "Display State In"=w322) -> ("state changed"=w316:bool, "Display State Out"=w323:T2)  [unwired: 5 in, 1 out]
              }
            }
            n91 = And(x=w294, y=w296) -> (x .and. y?=w295:bool)
            n92 = case shown="True" w295 {
              tunnel: w297 -> [_ w313]
              frame False {
              }
              frame True {
                n93 = property class="Tbl"(reference=w313, "Key Focus"=FALSE) -> (reference out=w312:refnum<vi>)  [unwired: 1 in, 1 out]
                n94 = property class="Tbl"(reference=w312, "Key Focus"=TRUE) -> ()  [unwired: 1 in, 2 out]
              }
            }
          }
          frame "Snap C to Peak" {
            n95 = Unbundle By Name(w338) -> ("Measurement Cursor Configuration.sideband.X center (C)"=w335:dbl)
            n96 = call-dynamic "Read Spectra from Data Object.vi"("component"=w324, "Data in"=w328) -> ("spectra info"=w329:T15[], "spectra"=w330:cluster{"x0":dbl, "dx":dbl, "Y":dbl[]}[], "Data out"=w327:T7)  [unwired: 5 in, 2 out]
            n97 = Index Array(array=w330) -> (element=w326:cluster{"x0":dbl, "dx":dbl, "Y":dbl[]})  [unwired: 1 in]
            n98 = Index Array(array=w329) -> (element=w325:T15)  [unwired: 1 in]
            n99 = Multiply(x=w335, y=cluster{"start":dbl, "stop":dbl} {"start"=0.9, "stop"=1.1} ("range")) -> (x*y=w333:cluster{"start":dbl, "stop":dbl})
            n100 = call-poly <vilib>:"SVFA Get Spectrum Subset.vi"("spectrum"=w326, "range"=w333, "spectrum info"=w325) -> ("spectrum subset"=w343:cluster{"x0":dbl, "dx":dbl, "magnitude":dbl[]}, "dup spectrum info"=w341:T15, "error out"=w340:errorcluster)  [unwired: 11 in, 3 out]
            n101 = call-poly <vilib>:"SVFA Spectrum Peak Search.vi"("spectrum"=w343, "peak search settings"=T10 {"single/multiple"=enum."Single Max Peak", "threshold"=inf}, "spectrum info in"=w341, "error in (no error)"=w340) -> ("peaks"=w337:cluster{"freq. or order":dbl, "value":dbl}[], "number of peaks"=w332:i32)  [unwired: 11 in, 3 out]
            n102 = case shown="1" w332 {
              tunnel: [w344 w352] -> w339
              tunnel: w338 -> [w344 w351]
              tunnel: w337 -> [_ w350]
              tunnel: w336 -> [_ w347]
              tunnel: [_ w345] -> w331
              frame 0, Default {
              }
              frame 1 {
                n103 = Index Array(array=w350) -> (element=w349:cluster{"freq. or order":dbl, "value":dbl})  [unwired: 1 in]
                n104 = Unbundle By Name(w349) -> ("freq. or order"=w348:dbl)
                n105 = call <vilib>:"Move Set on Cursor Move.vi"("Cursor.Position.X"=w348, "Cursor Name"="C", "Refnums for Resizing and Alignment"=w347, "Display State In"=w351) -> ("state changed"=w345:bool, "Display State Out"=w352:T2)  [unwired: 5 in, 1 out]
              }
            }
          }
          frame "Lock Band Cursor Span" {
            n106 = Unbundle By Name(w356) -> ("Measurement Cursor Configuration.band.B2"=w357:dbl, "Measurement Cursor Configuration.band.B1"=w358:dbl, "Measurement Cursor Configuration.band.Fixed bandwidth (B2-B1)"=w359:dbl)
            n107 = Subtract(x=w357, y=w358) -> (x-y=w363:dbl)
            n108 = Greater Than 0?(x=w359) -> (x > 0?=w360:bool)
            n109 = Negate(x=w363) -> (-x=w361:dbl)
            n110 = Select(t=w361, s=w360, f=w363) -> (s? t:f=w362:dbl)
            n111 = Bundle By Name(cluster=w356, "Measurement Cursor Configuration.band.Fixed bandwidth (B2-B1)"=w362) -> (w355:T2)
          }
          frame "Extended Bandwidth: 0.45*Fs", "Nyquist Bandwidth: 0.5*Fs", "Traditional Bandwidth: 0.39*Fs" {
            n112 = case shown="\"Nyquist Bandwidth: 0.5*Fs\", Default" w380 {
              tunnel: [w382 0.45 ("y") 0.5 ("y")] -> w377
              frame "Traditional Bandwidth: 0.39*Fs" {
                w382 = 0.390625  # 1/2.56
              }
              frame "Extended Bandwidth: 0.45*Fs" {
              }
              frame "Nyquist Bandwidth: 0.5*Fs", Default {
              }
            }
            n113 = call-dynamic "Read Spectra from Data Object.vi"("component"=w365, "Data in"=w369) -> ("spectra info"=w370:T15[], "spectra"=w371:cluster{"x0":dbl, "dx":dbl, "Y":dbl[]}[], "Data out"=w368:T7)  [unwired: 5 in, 2 out]
            n114 = Unbundle By Name(w375) -> ("Controls.Graph"=w374:refnum<vi>)
            n115 = Index Array(array=w371) -> (element=w367:cluster{"x0":dbl, "dx":dbl, "Y":dbl[]})  [unwired: 1 in]
            n116 = Index Array(array=w370) -> (element=w366:T15)  [unwired: 1 in]
            n117 = Unbundle By Name(w366) -> ("spectral info.window size"=w379:i32)
            n118 = Unbundle By Name(w367) -> ("dx"=w378:dbl)
            n119 = Multiply(x=w378, y=w379) -> (x*y=w376:dbl)
            n120 = Multiply(x=w376, y=w377) -> (x*y=w372:dbl)
            n121 = property class="WFGraph (strict)"(reference=w374, "XScale.ScaleFit"=u8 0 ("X Scale.Scale Fit"), "XScale.Maximum"=w372) -> ()  [unwired: 1 in, 2 out]
          }
          frame "Phase.-180to180", "Phase.-360to0", "Phase.0to360", "Phase.Unwrap" {
            n122 = case shown="\"Phase.-180to180\"" w386 {
              tunnel: [T11."No change" ("desired wrapping") T11."Unwrap" ("desired wrapping") T11."Wrap: -360 to 0" ("desired wrapping") T11."Wrap: -180 to 180" ("desired wrapping") T11."Wrap: 0 to 360" ("desired wrapping")] -> w385
              frame Default {
              }
              frame "Phase.Unwrap" {
              }
              frame "Phase.-360to0" {
              }
              frame "Phase.-180to180" {
              }
              frame "Phase.0to360" {
              }
            }
            n123 = Bundle By Name(cluster=w388, "phase spectrum view.desired wrapping"=w385) -> (w387:T2)
          }
          frame "Scaling.Cycles", "Scaling.Degrees", "Scaling.Radians" {
            n124 = case shown="\"Scaling.Radians\"" w401 {
              tunnel: [T12."Degrees" ("desired units") T12."Radians" ("desired units") T12."Cycles" ("desired units") T12."No change" ("desired units")] -> w398
              frame "Scaling.Degrees" {
              }
              frame "Scaling.Radians" {
              }
              frame "Scaling.Cycles" {
              }
              frame Default {
              }
            }
            n125 = Bundle By Name(cluster=w400, "phase spectrum view.desired units"=w398) -> (w399:T2)
          }
        }
        n126 = case shown="True" w107 {
          selector: w107 -> [_ w124]
          tunnel: w115 -> [w119 w127]
          tunnel: [w119 w126] -> w114
          tunnel: w106 -> [_ w122]
          tunnel: w113 -> [w118 w125]
          tunnel: [w118 w123] -> w112
          tunnel: [w117 w120] -> w111
          tunnel: w110 -> [w117 w121]
          frame False {
          }
          frame True {
            n127 = case shown="\"APP_SC_CLEAR_GRAPH\"" w122 {
              selector: w122 -> [w129 w136]
              tunnel: w127 -> [w133 w141]
              tunnel: [w132 w140] -> w126
              tunnel: w125 -> [w128 w139]
              tunnel: w124 -> [w134 w138]
              tunnel: [w128 w137] -> w123
              tunnel: w121 -> [w131 w135]
              tunnel: [w130 w135] -> w120
              frame "APP_SC_CLEAR_GRAPH" {
                n128 = Generate User Event(user event=w131, event data cluster=w134) -> (user event out=w130:refnum<user-event>)  [unwired: 2 in, 1 out]
                n129 = Bundle By Name(cluster=w133, "Action Name"=w129, "Data Changed?"=w134) -> (w132:T1)
              }
              frame Default {
                n130 = Generate User Event(user event=w139, event data cluster=w138) -> (user event out=w137:refnum<user-event>)  [unwired: 2 in, 1 out]
                n131 = Bundle By Name(cluster=w141, "Action Name"=w136, "State Changed?"=w138) -> (w140:T1)
              }
            }
          }
        }
      }
      event Pane Size {
        w410 = 10  # width - hidden splitter position
        w427 = TRUE
        n132 = event-data() -> ()  [unwired: 1 in, 1 out]
        n133 = Unbundle By Name(w412) -> ("Panes.Container"=w418:refnum<vi>, "Splitters.Moveable"=w419:refnum<vi>)
        n134 = property class="Ctl"(reference=w418) -> ("Width"=w421:u32)  [unwired: 1 in, 2 out]
        n135 = property class="Splitter"(reference=w419) -> ("Position"=w413:i32)  [unwired: 1 in, 2 out]
        n136 = Generate User Event(user event=w423, event data cluster=w427) -> (user event out=w422:refnum<user-event>)  [unwired: 2 in, 1 out]
        n137 = Bundle By Name(cluster=w426, "Action Name"="Resize", "State Changed?"=w427) -> (w425:T1)
        n138 = To Long Integer(number=w421) -> (32bit integer=w420:i32)
        n139 = Unbundle By Name(w411) -> ("View Table"=w415:bool)
        n140 = Subtract(x=w420, y=w410) -> (x-y=w417:i32)
        n141 = Not Equal?(x=w417, y=w413) -> (x != y?=w416:bool)
        n142 = And(x=w415, y=w416) -> (x .and. y?=w414:bool)
        n143 = case shown="True" w414 {
          tunnel: w411 -> [w430 w433]
          tunnel: [w430 w432] -> w408
          tunnel: w413 -> [_ w431]
          frame False {
          }
          frame True {
            n144 = Bundle By Name(cluster=w433, "Moveable Splitter Position"=w431) -> (w432:T2)
          }
        }
      }
      event "View Table": Value Change {
        w443 = TRUE
        n145 = event-data() -> ("NewVal"=w435:bool)  [unwired: 1 in]
        n146 = Bundle By Name(cluster=w437, "View Table"=w435) -> (w436:T2)
        n147 = Generate User Event(user event=w439, event data cluster=w443) -> (user event out=w438:refnum<user-event>)  [unwired: 2 in, 1 out]
        n148 = Bundle By Name(cluster=w442, "Action Name"="View Table Value Change", "State Changed?"=w443) -> (w441:T1)
      }
      event "Spectra Graph": Autoscale Range Change {
        n149 = event-data() -> ("Kind"=w453:enum16{"X-Scale", "Y-Scale", "Z-Scale"}, "ScaleRef"=w452:refnum<vi>)  [unwired: 1 in]
        n150 = property class="GrphScl"(reference=w452) -> ("ScaleFit"=w451:u8)  [unwired: 1 in, 2 out]
        n151 = case shown="\"Y-Scale\"" w453 {
          tunnel: w448 -> [w459 w461]
          tunnel: [w459 w460] -> w447
          tunnel: [w458 w464] -> w449
          tunnel: w450 -> [w458 w463]
          tunnel: w451 -> [_ w462]
          frame "X-Scale", Default {
          }
          frame "Y-Scale" {
            n152 = case shown="1, 2" w462 {
              tunnel: w461 -> [w465 w471]
              tunnel: w463 -> [w466 w467]
              tunnel: [w465 w468] -> w460
              tunnel: [w466 w467] -> w464
              frame 0, Default {
                # "YScaleFit\nManual"
              }
              frame 1, 2 {
                # "YScaleFit\nAuto"
                n153 = call <vilib>:"Defer Panel Updates.vi"("Refnums for FP Objects"=w467, "State in"=w471) -> ("State out"=w470:T2)  [unwired: 8 in, 1 out]
                n154 = call <vilib>:"Adjust Cursor Y Position to Maintain Label Placement.vi"("Refnums for Resizing and Alignment"=w467, "Display State In"=w470) -> ("Display State Out"=w469:T2)  [unwired: 9 in]
                n155 = call <vilib>:"UnDefer Panel Updates.vi"("Refnums for FP Objects"=w467, "State in"=w469) -> ("State out"=w468:T2)  [unwired: 8 in, 1 out]
              }
            }
          }
        }
      }
      event "Spectra Graph": Scale Range Change {
        (unwired) "Scale Range Change"
        # "this tells us if the scale range changed due to autoscale being set"
        n156 = event-data() -> ("Kind"=w477:enum16{"X-Scale", "Y-Scale", "Z-Scale"}, "ScaleRef"=w481:refnum<vi>)  [unwired: 1 in]
        n157 = case shown="0" w473 {
          selector: w473 -> [_ w485]
          tunnel: w481 -> [_ w487]
          tunnel: [_ w486] -> w476
          tunnel: [u8 0 ("Scale Fit") w485] -> w472
          frame Default {
          }
          frame 0 {
            n158 = property class="GrphScl"(reference=w487, "ScaleFit"=w485) -> (error out=w486:errorcluster)  [unwired: 1 in, 1 out]
          }
        }
        n159 = case shown="\"Y-Scale\"" w477 {
          tunnel: w480 -> [_ w489]
          tunnel: w479 -> [w488 w493]
          tunnel: [w488 w490] -> w478
          tunnel: w476 -> [_ _]
          frame Default {
          }
          frame "Y-Scale" {
            n160 = call <vilib>:"Defer Panel Updates.vi"("Refnums for FP Objects"=w489, "State in"=w493) -> ("State out"=w492:T2)  [unwired: 8 in, 1 out]
            n161 = call <vilib>:"Adjust Cursor Y Position to Maintain Label Placement.vi"("Refnums for Resizing and Alignment"=w489, "Display State In"=w492) -> ("Display State Out"=w491:T2)  [unwired: 9 in]
            n162 = call <vilib>:"UnDefer Panel Updates.vi"("Refnums for FP Objects"=w489, "State in"=w491) -> ("State out"=w490:T2)  [unwired: 8 in, 1 out]
          }
        }
      }
      event "Spectra Graph": Cursor Move; "Spectra Graph": Cursor Grab {
        n163 = event-data() -> ("CursRef"=w505:refnum<vi>, "CursLoc"=w506:cluster{"X":dbl, "Y":dbl})  [unwired: 1 in]
        n164 = property class="Curs"(reference=w505) -> ("Cursor Name"=w504:string)  [unwired: 1 in, 2 out]
        n165 = Unbundle By Name(w506) -> ("X"=w503:dbl)
        n166 = call <vilib>:"Move Set on Cursor Move.vi"("Cursor.Position.X"=w503, "Cursor Name"=w504, "Refnums for Resizing and Alignment"=w502, "Display State In"=w514) -> ("cursor type"=w496:string, "state changed"=w495:bool, "Display State Out"=w498:T2)  [unwired: 5 in]
        n167 = call <vilib>:"Conditionally Unlock 1X Cursor.vi"("cursor type"=w496, "state changed in"=w495, "Display State Out in"=w498) -> ("state changed out"=w494:bool, "Display State Out out"=w497:T2)  [unwired: 7 in]
        n168 = Unbundle By Name(w502) -> ("Controls.Focus Boolean"=w501:refnum<vi>)
        n169 = property class="Bool (strict)"(reference=w501, "Key Focus"=TRUE) -> ()  [unwired: 1 in, 2 out]
        n170 = case shown="True" w494 {
          selector: w494 -> [_ w521]
          tunnel: w513 -> [w518 w525]
          tunnel: [w518 w524] -> w512
          tunnel: "Cursor Move" -> [_ w523]
          tunnel: w510 -> [w517 w522]
          tunnel: [w517 w520] -> w509
          tunnel: [w516 w519] -> w508
          tunnel: w507 -> [w516 w519]
          frame False {
          }
          frame True {
            n171 = Generate User Event(user event=w522, event data cluster=w521) -> (user event out=w520:refnum<user-event>)  [unwired: 2 in, 1 out]
            n172 = Bundle By Name(cluster=w525, "Action Name"=w523, "State Changed?"=w521) -> (w524:T1)
          }
        }
      }
      event "Spectra Graph": Plot Attribute Change {
        n173 = event-data() -> ()  [unwired: 1 in, 2 out]
        n174 = call <vilib>:"Update State Plot Properties.vi"("Refnums for FP Objects"=w527, "State in"=w529) -> ("State out"=w528:T2)  [unwired: 9 in]
      }
      event "Cursor Table": Value Change {
        n175 = event-data() -> ("NewVal"=w547:string[][], "OldVal"=w535:string[][], "CtlRef"=w536:refnum<vi>)  [unwired: 1 in]
        n176 = call <vilib>:"Verify New Value is Valid X.vi"("OldVal"=w535, "NewVal"=w547, "Refnums for Resizing and Alignment"=w540, "State in"=w542) -> ("X position"=w537:dbl, "cursor name"=w538:string, "Refnums for Resizing and Alignment out"=w539:T8, "State out"=w541:T2, "valid X change"=w544:bool)  [unwired: 3 in]
        n177 = case shown="True" w544 {
          selector: w544 -> [w555 _]
          tunnel: w539 -> [_ w565]
          tunnel: w541 -> [w556 w564]
          tunnel: [w556 w560] -> w545
          tunnel: [w555 w557] -> w543
          tunnel: w538 -> [_ w563]
          tunnel: w537 -> [_ w562]
          frame False {
          }
          frame True {
            n178 = call <vilib>:"Move Set on Cursor Move.vi"("Cursor.Position.X"=w562, "Cursor Name"=w563, "Refnums for Resizing and Alignment"=w565, "Display State In"=w564) -> ("cursor type"=w558:string, "state changed"=w559:bool, "Display State Out"=w561:T2)  [unwired: 5 in]
            n179 = call <vilib>:"Conditionally Unlock 1X Cursor.vi"("cursor type"=w558, "state changed in"=w559, "Display State Out in"=w561) -> ("state changed out"=w557:bool, "Display State Out out"=w560:T2)  [unwired: 7 in]
          }
        }
        n180 = case shown="False" w543 {
          selector: w543 -> [_ w571]
          tunnel: w553 -> [w570 w577]
          tunnel: [w570 w576] -> w552
          tunnel: "Cursor Table Value Change" -> [_ w575]
          tunnel: w551 -> [w569 w574]
          tunnel: [w569 w573] -> w550
          tunnel: [w568 w572] -> w549
          tunnel: w548 -> [w568 w572]
          tunnel: w536 -> [w567 _]
          tunnel: w535 -> [w566 _]
          frame False {
            n181 = property on="Property Node" class="Tbl (strict)"(reference=w567, "Value"=w566) -> ()  [unwired: 1 in, 2 out]
          }
          frame True {
            n182 = Bundle By Name(cluster=w577, "State Changed?"=w571, "Action Name"=w575) -> (w576:T1)
            n183 = Generate User Event(user event=w574, event data cluster=w571) -> (user event out=w573:refnum<user-event>)  [unwired: 2 in, 1 out]
          }
        }
      }
      event "Cursor Table", "Focus Boolean": Key Down? {
        n184 = event-data() -> ("VKey"=w588:T21, "PlatMods"=w581:T22)  [unwired: 1 in]
        n185 = call <vilib>:"Update Control Based on Key Down.vi"("PlatMods"=w581, "VKey"=w588, "Refnums for Resizing and Alignment in"=w585, "display state in"=w587) -> ("Position.X"=w582:dbl, "selected cursor"=w583:string, "Refnums for Resizing and Alignment out"=w584:T8, "display state out"=w586:T2, "discard?"=w579:bool)  [unwired: 3 in]
        n186 = case shown="True" w579 {
          selector: w579 -> [w598 _]
          tunnel: w584 -> [_ w608]
          tunnel: w586 -> [w599 w607]
          tunnel: [w599 w603] -> w589
          tunnel: [w598 w600] -> w580
          tunnel: w583 -> [_ w606]
          tunnel: w582 -> [_ w605]
          frame False {
          }
          frame True {
            n187 = call <vilib>:"Move Set on Cursor Move.vi"("Cursor.Position.X"=w605, "Cursor Name"=w606, "Refnums for Resizing and Alignment"=w608, "Display State In"=w607) -> ("cursor type"=w601:string, "state changed"=w602:bool, "Display State Out"=w604:T2)  [unwired: 5 in]
            n188 = call <vilib>:"Conditionally Unlock 1X Cursor.vi"("cursor type"=w601, "state changed in"=w602, "Display State Out in"=w604) -> ("state changed out"=w600:bool, "Display State Out out"=w603:T2)  [unwired: 7 in]
          }
        }
        n189 = case shown="True" w580 {
          selector: w580 -> [_ w612]
          tunnel: w596 -> [w611 w618]
          tunnel: [w611 w617] -> w595
          tunnel: "Cursor Move" -> [_ w616]
          tunnel: w594 -> [w610 w615]
          tunnel: [w610 w614] -> w593
          tunnel: [w609 w613] -> w592
          tunnel: w591 -> [w609 w613]
          frame False {
          }
          frame True {
            n190 = Bundle By Name(cluster=w618, "State Changed?"=w612, "Action Name"=w616) -> (w617:T1)
            n191 = Generate User Event(user event=w615, event data cluster=w612) -> (user event out=w614:refnum<user-event>)  [unwired: 2 in, 1 out]
          }
        }
        n192 = event-data("Discard?"=w579) -> ()  [unwired: 1 in, 1 out]
      }
      event "Cursor Table", "Focus Boolean": event type 3.0.x8000000b {
        n193 = event-data() -> ("VKey"=w624:T21, "PlatMods"=w625:T22)  [unwired: 1 in]
        n194 = call <vilib>:"Update Control Based on Key Down.vi"("PlatMods"=w625, "VKey"=w624, "Refnums for Resizing and Alignment in"=w627, "display state in"=w628) -> ("Position.X"=w620:dbl, "selected cursor"=w621:string, "Refnums for Resizing and Alignment out"=w622:T8, "display state out"=w623:T2, "discard?"=w626:bool)  [unwired: 3 in]
        n195 = case shown="True" w626 {
          selector: w626 -> [w639 _]
          tunnel: w622 -> [_ w649]
          tunnel: w623 -> [w640 w648]
          tunnel: [w640 w642] -> w630
          tunnel: [w639 w641] -> w629
          tunnel: w621 -> [_ w647]
          tunnel: w620 -> [_ w646]
          frame False {
          }
          frame True {
            n196 = call <vilib>:"Move Set on Cursor Move.vi"("Cursor.Position.X"=w646, "Cursor Name"=w647, "Refnums for Resizing and Alignment"=w649, "Display State In"=w648) -> ("cursor type"=w644:string, "state changed"=w645:bool, "Display State Out"=w643:T2)  [unwired: 5 in]
            n197 = call <vilib>:"Conditionally Unlock 1X Cursor.vi"("cursor type"=w644, "state changed in"=w645, "Display State Out in"=w643) -> ("state changed out"=w641:bool, "Display State Out out"=w642:T2)  [unwired: 7 in]
          }
        }
        n198 = case shown="True" w629 {
          selector: w629 -> [_ w653]
          tunnel: w637 -> [w652 w659]
          tunnel: [w652 w658] -> w636
          tunnel: "Cursor Move" -> [_ w657]
          tunnel: w635 -> [w651 w656]
          tunnel: [w651 w655] -> w634
          tunnel: [w650 w654] -> w633
          tunnel: w632 -> [w650 w654]
          frame False {
          }
          frame True {
            n199 = Bundle By Name(cluster=w659, "State Changed?"=w653, "Action Name"=w657) -> (w658:T1)
            n200 = Generate User Event(user event=w656, event data cluster=w653) -> (user event out=w655:refnum<user-event>)  [unwired: 2 in, 1 out]
          }
        }
        n201 = event-data("Discard?"=w626) -> ()  [unwired: 1 in, 1 out]
      }
      event "Cursor Table": Mouse Down {
        (unwired) "Cursor Table Mouse Down" ("ItemTag")
        n202 = event-data() -> ("Coords.Horizontal"=w664:i32, "Coords.Vertical"=w663:i32)  [unwired: 1 in]
        n203 = Bundle By Name(cluster=cluster{"horizontal":i32, "vertical":i32} {"horizontal"=0, "vertical"=0} ("Point"), "horizontal"=w664, "vertical"=w663) -> (w661:cluster{"horizontal":i32, "vertical":i32})
        n204 = call <vilib>:"Set Active Cursor from Table.vi"("Point"=w661, "Refnums for Resizing and Alignment"=w667, "Display State In"=w666) -> ("Display State Out"=w665:T2)  [unwired: 8 in]
      }
      event Display State Change; User Event {
        w678 = T13 "Display State Change"
        # "Display State changed as a result of dropping a new instance of this XControl, copying, undoing an operation or executing a custom property or method on this XControl. Update the appearance accordingly."
        n205 = event-data() -> ()  [unwired: 1 in, 3 out]
        n206 = property class="Data.lvclass"(reference=w674) -> (reference out=w673:T7, "Properties:Number of Channels"=w672:i32)  [unwired: 1 in, 1 out]
        n207 = Unbundle By Name(w680) -> ("Action Name"=w683:string)
        n208 = case shown="Default" w683 {
          selector: w683 -> [_ _ w713]
          tunnel: [w702 w704 w706] -> w687
          tunnel: w685 -> [w702 w704 w709]
          tunnel: w684 -> [w701 w703 w710]
          tunnel: [w701 w703 w710] -> w682
          tunnel: [TRUE ("Data Changed?") _ w712] -> w675
          tunnel: w672 -> [_ _ w705]
          frame "Cursor Move", "Lock 1X to Peak", "Snap 1X to Peak" {
          }
          frame "1X Cursor Track" {
          }
          frame Default {
            n209 = call <vilib>:"Defer Panel Updates.vi"("Refnums for FP Objects"=w710, "State in"=w709) -> ("State out"=w707:T2)  [unwired: 8 in, 1 out]
            n210 = call <vilib>:"Update Graph Cursors from State.vi"("Refnums for FP Objects"=w710, "State in"=w707) -> ("State out"=w714:T2)  [unwired: 9 in]
            n211 = call <vilib>:"Set Graph Scale Properties.vi"("Refnums in"=w710, "Display State In"=w714) -> ("Display State out"=w716:T2)  [unwired: 9 in]
            n212 = call <vilib>:"Resize and Align.vi"("number of channels"=w705, "Refnums for Resizing and Alignment"=w710, "State in"=w716) -> ("State out"=w715:T2)  [unwired: 7 in, 1 out]
            n213 = call <vilib>:"Adjust Cursor Y Position to Maintain Label Placement.vi"("Refnums for Resizing and Alignment"=w710, "Display State In"=w715) -> ("Display State Out"=w717:T2)  [unwired: 9 in]
            n214 = call <vilib>:"Set Colors.vi"("Refnums"=w710, "Display State In"=w717) -> ("Display State Out"=w708:T2)  [unwired: 9 in]
            n215 = Not Equal?(x="Resize", y=w713) -> (x != y?=w712:bool)
            n216 = call <vilib>:"UnDefer Panel Updates.vi"("Refnums for FP Objects"=w710, "State in"=w708) -> ("State out"=w706:T2)  [unwired: 8 in, 1 out]
          }
        }
        n217 = case shown="True" w675 {
          selector: w675 -> [_ w693]
          tunnel: w689 -> [w691 w699]
          tunnel: [w691 w698] -> w688
          tunnel: w680 -> [w690 w697]
          tunnel: [w690 w696] -> w679
          tunnel: w678 -> [_ w695]
          tunnel: [w692 w694] -> w676
          tunnel: w677 -> [w692 w694]
          frame False {
          }
          frame True {
            n218 = Bundle By Name(cluster=w697, "Action Name"=w695, "Data Changed?"=w693) -> (w696:T1)
            n219 = Generate User Event(user event=w699, event data cluster=w693) -> (user event out=w698:refnum<user-event>)  [unwired: 2 in, 1 out]
          }
        }
        n220 = call <vilib>:"Generate Matching User Event.vi"("event"=w678, "Display State in"=w687) -> ("Display State out"=w686:T2)  [unwired: 8 in, 1 out]
      }
      event Data Change; User Event {
        # "A value was written to the XControl's terminal, local or value property.\nUpdate the appearance in response to data change."
        n221 = event-data() -> ()  [unwired: 1 in, 1 out]
        n222 = Unbundle By Name(w719) -> ("Action Name"=w718:string)
        n223 = case shown="\"APP_SC_CLEAR_GRAPH\"" w718 {
          selector: w718 -> [w742 _]
          tunnel: w735 -> [w741 w748]
          tunnel: [w740 w747] -> w734
          tunnel: [w743 w755] -> w731
          tunnel: [w737 w762] -> w730
          tunnel: w728 -> [w743 w759]
          tunnel: [_ w758] -> w727
          tunnel: w721 -> [w737 w757]
          tunnel: [w742 w754] -> w720
          frame "APP_SC_CLEAR_GRAPH" {
            n224 = Unbundle By Name(w737) -> ("spectrum component"=w736:T5)
            n225 = call-dynamic "Read Spectra from Data Object.vi"("component"=w736, "Data in"=w741) -> ("spectra"=w739:cluster{"x0":dbl, "dx":dbl, "Y":dbl[]}[], "Data out"=w740:T7)  [unwired: 5 in, 3 out]
            n226 = local write "Spectra Graph"(w739) -> ()
            n227 = local write "Cursor Table"(string[][] [[" "]] ("Cursor Table")) -> ()
          }
          frame Default {
            n228 = Unbundle By Name(w757) -> ("spectrum component"=w746:T5, "desired spectrum view.scaling"=w763:T23, "desired spectrum view.spectral density"=w764:T9)
            n229 = Unbundle By Name(w757) -> ("Measurement Cursor Configuration.harmonic.enable harmonics"=w751:bool, "Lock 1X to Peak"=w756:bool, "View Table"=w753:bool, "Measurement Cursor Configuration.harmonic.X reference (1X)"=w749:dbl)
            n230 = call-dynamic "Read Spectra from Data Object.vi"("component"=w746, "Data in"=w748) -> ("spectra info"=w744:T15[], "spectra"=w745:cluster{"x0":dbl, "dx":dbl, "Y":dbl[]}[], "Data out"=w747:T7)  [unwired: 5 in, 2 out]
            n231 = Greater Than 0?(x=w749) -> (x > 0?=w750:bool)
            n232 = case shown="32, 37" w746 {
              tunnel: w764 -> [_ w789 _ _]
              tunnel: w763 -> [_ w788 _ _]
              tunnel: [w768 w787 w841 w862] -> w761
              tunnel: [w765 w772 w842 w858] -> w760
              tunnel: w759 -> [w767 w786 w848 w863]
              tunnel: w749 -> [_ w776 _ _]
              tunnel: [_ w785 _ _] -> w758
              tunnel: w757 -> [w768 w784 w841 w862]
              tunnel: w756 -> [_ w779 _ _]
              tunnel: [w767 w783 w847 w861] -> w755
              tunnel: [_ w782 _ _] -> w754
              tunnel: w753 -> [_ w781 w846 w860]
              tunnel: [w766 w773 w844 w859] -> w752
              tunnel: w751 -> [_ w780 _ _]
              tunnel: w750 -> [_ w777 _ _]
              tunnel: w745 -> [w766 w770 w838 w859]
              tunnel: w744 -> [w765 w769 w837 w858]
              frame Default {
              }
              frame 32, 37 {
                n233 = case shown="True" w777 {
                  tunnel: [cluster{"start":dbl, "stop":dbl} {"start"=-1.0, "stop"=-1.0} w793] -> w771
                  tunnel: w776 -> [_ w791]
                  frame False {
                  }
                  frame True {
                    n234 = Multiply(x=cluster{"start":dbl, "stop":dbl} {"start"=0.5, "stop"=1.5} ("range"), y=w791) -> (x*y=w793:cluster{"start":dbl, "stop":dbl})
                  }
                }
                n235 = And(x=w780, y=w779) -> (x .and. y?=w778:bool)
                n236 = call-poly <vilib>:"SVFA Unit Conversion.vi"("spectra"=w770, "desired scaling"=w788, "spectral density desired"=w789, "spectrum info in"=w769) -> ("converted spectra"=w775:cluster{"x0":dbl, "dx":dbl, "magnitude":dbl[]}[], "spectrum info out"=w774:T15[])  [unwired: 12 in, 2 out]
                n237 = case shown="True" w778 {
                  tunnel: [w799 w817] -> w787
                  tunnel: w786 -> [w798 w814]
                  tunnel: [_ w816] -> w785
                  tunnel: w784 -> [w799 w815]
                  tunnel: [w797 w812] -> w783
                  tunnel: [_ w813] -> w782
                  tunnel: w781 -> [w796 _]
                  tunnel: w775 -> [w795 w811]
                  tunnel: w774 -> [w794 w810]
                  tunnel: [w795 w811] -> w773
                  tunnel: [w794 w810] -> w772
                  tunnel: w771 -> [_ w809]
                  frame False {
                    n238 = case shown="False" w796 {
                      tunnel: w798 -> [w800 w801]
                      tunnel: [w800 w801] -> w797
                      frame False {
                      }
                      frame True {
                        n239 = Unbundle By Name(w801) -> ("Controls.Table"=w804:refnum<vi>)
                        n240 = property class="Tbl"(reference=w804) -> (reference out=w802:refnum<vi>, "Key Focus"=w803:bool)  [unwired: 1 in, 1 out]
                        n241 = case shown="True" w803 {
                          tunnel: w802 -> [_ w807]
                          frame False {
                          }
                          frame True {
                            n242 = property class="Tbl"(reference=w807, "Key Focus"=FALSE) -> (reference out=w806:refnum<vi>)  [unwired: 1 in, 1 out]
                            n243 = property class="Tbl"(reference=w806, "Key Focus"=TRUE) -> ()  [unwired: 1 in, 2 out]
                          }
                        }
                      }
                    }
                  }
                  frame True {
                    n244 = Index Array(array=w810) -> (element=w819:T15)  [unwired: 1 in]
                    n245 = Index Array(array=w811) -> (element=w818:cluster{"x0":dbl, "dx":dbl, "magnitude":dbl[]})  [unwired: 1 in]
                    n246 = call-poly <vilib>:"SVFA Get Spectrum Subset.vi"("spectrum"=w818, "range"=w809, "spectrum info"=w819) -> ("spectrum subset"=w820:cluster{"x0":dbl, "dx":dbl, "magnitude":dbl[]}, "dup spectrum info"=w822:T15, "error out"=w823:errorcluster)  [unwired: 11 in, 3 out]
                    n247 = call-poly <vilib>:"SVFA Spectrum Peak Search.vi"("spectrum"=w820, "peak search settings"=T10 {"single/multiple"=enum."Single Max Peak", "threshold"=inf}, "spectrum info in"=w822, "error in (no error)"=w823) -> ("peaks"=w824:cluster{"freq. or order":dbl, "value":dbl}[], "number of peaks"=w825:i32)  [unwired: 11 in, 3 out]
                    n248 = case shown="1" w825 {
                      tunnel: [w827 w836] -> w817
                      tunnel: w815 -> [w827 w835]
                      tunnel: w824 -> [_ w834]
                      tunnel: w814 -> [w826 w828]
                      tunnel: [_ w830] -> w816
                      tunnel: [_ "1X Cursor Track"] -> w813
                      tunnel: [w826 w828] -> w812
                      frame 0, Default {
                      }
                      frame 1 {
                        n249 = Index Array(array=w834) -> (element=w833:cluster{"freq. or order":dbl, "value":dbl})  [unwired: 1 in]
                        n250 = Unbundle By Name(w833) -> ("freq. or order"=w832:dbl)
                        n251 = call <vilib>:"Move Set on Cursor Move.vi"("Cursor.Position.X"=w832, "Cursor Name"="1X", "Refnums for Resizing and Alignment"=w828, "Display State In"=w835) -> ("state changed"=w830:bool, "Display State Out"=w836:T2)  [unwired: 5 in, 1 out]
                      }
                    }
                  }
                }
              }
              frame 33 {
                n252 = Unbundle By Name(w841) -> ("phase spectrum view.desired wrapping"=w840:u16, "phase spectrum view.desired units"=w839:u16)
                n253 = case shown="True" w846 {
                  tunnel: w848 -> [w849 w850]
                  tunnel: [w849 w850] -> w847
                  frame False {
                  }
                  frame True {
                    n254 = Unbundle By Name(w850) -> ("Controls.Table"=w853:refnum<vi>)
                    n255 = property class="Tbl"(reference=w853) -> (reference out=w851:refnum<vi>, "Key Focus"=w852:bool)  [unwired: 1 in, 1 out]
                    n256 = case shown="True" w852 {
                      tunnel: w851 -> [_ w856]
                      frame False {
                      }
                      frame True {
                        n257 = property class="Tbl"(reference=w856, "Key Focus"=FALSE) -> (reference out=w855:refnum<vi>)  [unwired: 1 in, 1 out]
                        n258 = property class="Tbl"(reference=w855, "Key Focus"=TRUE) -> ()  [unwired: 1 in, 2 out]
                      }
                    }
                  }
                }
                n259 = call-poly <vilib>:"SVFA Wrap or Unwrap Phase.vi"("phase spectra in"=w838, "desired wrapping"=w840, "spectrum info"=w837) -> ("phase spectra out"=w845:cluster{"f0":dbl, "df":dbl, "phase":dbl[]}[], "dup spectrum info"=w843:T15[])  [unwired: 13 in, 2 out]
                n260 = call-poly <vilib>:"SVFA Phase Unit Conversion.vi"("phase spectra"=w845, "desired units"=w839, "spectrum info in"=w843) -> ("converted phase spectra"=w844:cluster{"x0":dbl, "dx":dbl, "phase":dbl[]}[], "spectrum info out"=w842:T15[])  [unwired: 13 in, 2 out]
              }
              frame 34..36 {
                n261 = case shown="True" w860 {
                  tunnel: w863 -> [w864 w865]
                  tunnel: [w864 w865] -> w861
                  frame False {
                  }
                  frame True {
                    n262 = Unbundle By Name(w865) -> ("Controls.Table"=w868:refnum<vi>)
                    n263 = property class="Tbl"(reference=w868) -> (reference out=w866:refnum<vi>, "Key Focus"=w867:bool)  [unwired: 1 in, 1 out]
                    n264 = case shown="True" w867 {
                      tunnel: w866 -> [_ w871]
                      frame False {
                      }
                      frame True {
                        n265 = property class="Tbl"(reference=w871, "Key Focus"=FALSE) -> (reference out=w870:refnum<vi>)  [unwired: 1 in, 1 out]
                        n266 = property class="Tbl"(reference=w870, "Key Focus"=TRUE) -> ()  [unwired: 1 in, 2 out]
                      }
                    }
                  }
                }
              }
            }
            "Spectra Graph" <- w752
            n267 = call <vilib>:"Get Cursor Values from Data.vi"("spectra"=w752, "spectra info"=w760, "Refnums for FP Objects"=w755, "Display State In"=w761) -> ("Display State Out"=w762:T2)  [unwired: 4 in, 3 out]
          }
        }
        n268 = case shown="True" w727 {
          selector: w727 -> [_ w876]
          tunnel: w719 -> [w875 w882]
          tunnel: [w875 w881] -> w724
          tunnel: w720 -> [_ w880]
          tunnel: w725 -> [w874 w879]
          tunnel: [w874 w878] -> w723
          tunnel: [w873 w877] -> w722
          tunnel: w726 -> [w873 w877]
          frame False {
          }
          frame True {
            n269 = Bundle By Name(cluster=w882, "State Changed?"=w876, "Action Name"=w880) -> (w881:T1)
            n270 = Generate User Event(user event=w879, event data cluster=w876) -> (user event out=w878:refnum<user-event>)  [unwired: 2 in, 1 out]
          }
        }
        n271 = call <vilib>:"Generate Matching User Event.vi"("event"=T13 "Data Change", "Display State in"=w730) -> ("Display State out"=w729:T2)  [unwired: 8 in, 1 out]
      }
      event Direction Change {
        (unwired) "Direction Change"
        # "The direction of the XControl changed from a control to an indicator or vice versa. Update the appearance accordingly."
        n272 = event-data() -> ()  [unwired: 1 in, 4 out]
        n273 = Unbundle By Name(w884) -> ("Splitters.Locked"=w890:refnum<vi>)
        n274 = Unbundle By Name(w894) -> ("Refnum"=w886:refnum<vi>)
        n275 = property class="Splitter"(reference=w890, "Colors"=T14 {"Foreground Color"=16777216, "Background Color"=16777216}) -> ()  [unwired: 1 in, 2 out]
        n276 = property class="Ctl"(reference=w886, "SyncDisp"=TRUE ("Synchronous Display")) -> ()  [unwired: 1 in, 2 out]
      }
      event Exec State Change {
        (unwired) "Exec State Change"
        # "The VI owning the XControl changed from Edit Mode  to Run Mode or vice versa.\nUpdate the appearance accordingly."
        # "Handle Edit Mode & Run Mode\ncase differently"
        n277 = event-data() -> ()  [unwired: 1 in, 4 out]
        n278 = Unbundle By Name(w902) -> ()  [unwired: 1 out]
      }
    }
  }
  "Display State Out" <- w5
  "Data Out" <- w7
  "Action" <- w2
